vi "Get Target Branch Names.vi"(8 "error in":errorcluster, 11 "Peer Review in":refnum<class "Peer Review.lvclass">) -> (0 "error out":errorcluster, 3 "Peer Review out":refnum<class "Peer Review.lvclass">)   [LabVIEW 2020, in "Peer Review.lvclass"]
uses:
  Peer Review.lvclass
  Peer Review.lvclass/Peer Review.ctl
  <vilib>/Utility/error.llb/Trim Whitespace One-Sided.vi
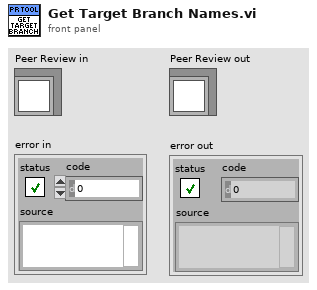
[diagram p1: front panel]
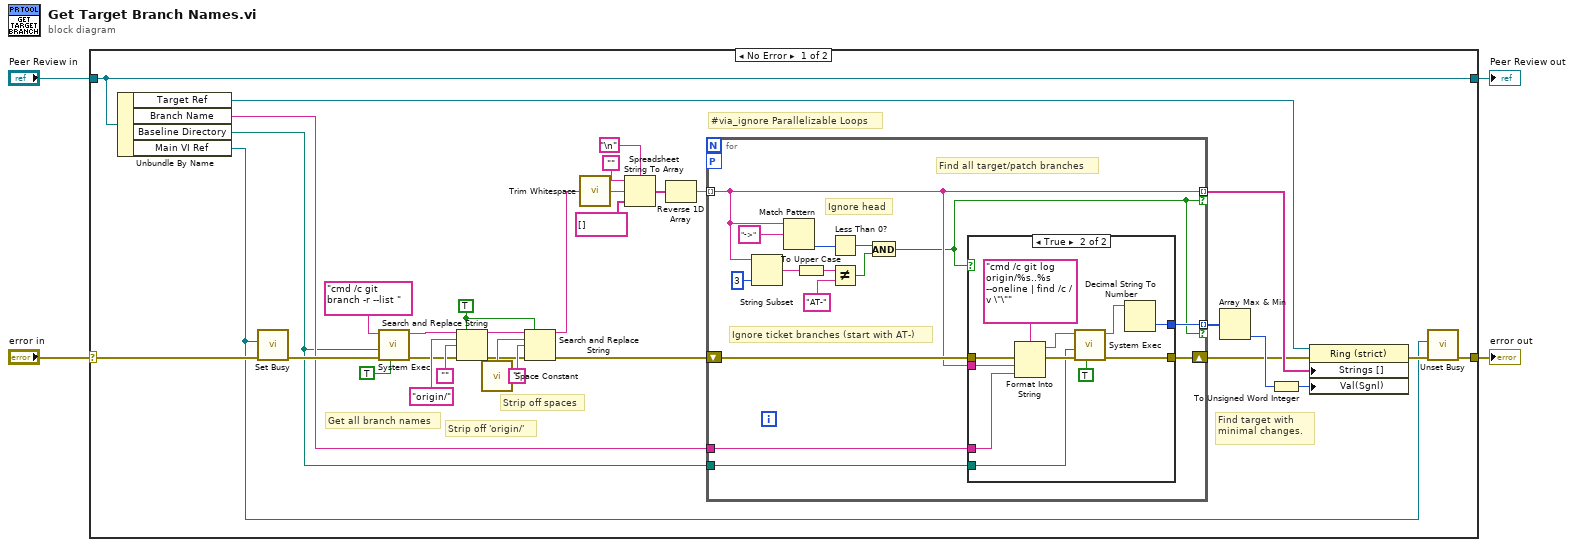
[diagram p0: block diagram]
diagram:
  n1 = case shown="No Error" "error in" {
    selector: "error in" -> [w33 w65]
    tunnel: [w31 w65] -> w3
    tunnel: [w37 w66] -> w4
    tunnel: "Peer Review in" -> [w37 w66]
    frame No Error {
      w11 = TRUE ("replace all? (F)")
      # "#via_ignore Parallelizable Loops"
      # "Find target with minimal changes."
      # "Strip off spaces"
      # "Strip off 'origin/'"
      # "Get all branch names"
      n2 = Unbundle By Name(w37) -> ("Target Ref"=w36:refnum<vi>, "Branch Name"=w8:string, "Baseline Directory"=w7:path, "Main VI Ref"=w10:refnum<vi>)
      n3 = call <vilib>:"Set Busy.vi"("error in (no error)"=w33, "VI reference (current VI)"=w10) -> ("error out"=w13:errorcluster)  [unwired: 8 in, 1 out]
      n4 = call <vilib>:"System Exec.vi"("run minimized? (F)"=TRUE, "error in (no error)"=w13, "working directory"=w7, "command line"="cmd /c git branch -r --list " ("String 2")) -> ("error out"=w21:errorcluster, "standard output"=w23:string)  [unwired: 4 in, 2 out]
      n5 = Search and Replace String(replace all?=w11, input string=w23, search string="origin/", replace string="" ("Empty String Constant"), error in=w21) -> (result string=w27:string, error out=w24:errorcluster)  [unwired: 3 in, 2 out]
      n6 = call <vilib>:"Space Constant.vi"() -> ("String"=w25:string)
      n7 = Search and Replace String(replace all?=w11, input string=w27, search string=w25, replace string="" ("Empty String Constant"), error in=w24) -> (result string=w16:string, error out=w9:errorcluster)  [unwired: 3 in, 2 out]
      n8 = call <vilib>:"Trim Whitespace.vi"("string"=w16) -> ("trimmed string"=w17:string)  [unwired: 1 in]
      n9 = Spreadsheet String To Array(delimiter (Tab)="\n" ("Line Feed Constant"), format string="", spreadsheet string=w17, array type (2D Dbl)=string[] [] ("Strings []")) -> (array=w15:string[])
      n10 = Reverse 1D Array(array=w15) -> (reversed array=w14:string[])
      n11 = for {
        tunnel: w14 -> [w40] mode=indexing
        tunnel: [w40] -> w12 mode=indexing if=w38
        workers-P: _ -> [_]
        tunnel: w8 -> [w50]
        tunnel: [w49] -> w6 mode=indexing if=w38
        tunnel: w7 -> [w48]
        shift-right: [w51] -> w5
        shift-left: w9 -> [w52]
        # "Ignore ticket branches (start with AT-)"
        # "Ignore head"
        # "Find all target/patch branches"
        n12 = String Subset(string=w40, length (rest)=3 ("length (rest)")) -> (substring=w44:string)  [unwired: 1 in]
        n13 = Match Pattern(string=w40, regular expression="->") -> (offset past match=w46:i32)  [unwired: 1 in, 3 out]
        n14 = To Upper Case(1:w44) -> (0:w43:string)
        n15 = Less Than 0?(x=w46) -> (x < 0?=w39:bool)
        n16 = Not Equal?(x=w43, y="AT-") -> (x != y?=w42:bool)
        n17 = And(x=w39, y=w42) -> (x .and. y?=w38:bool)
        n18 = case shown="True" w38 {
          tunnel: w52 -> [w53 w60]
          tunnel: [w53 w59] -> w51
          tunnel: w40 -> [_ w58]
          tunnel: w50 -> [_ w57]
          tunnel: [_ w54] -> w49
          tunnel: w48 -> [_ w55]
          frame False {
          }
          frame True {
            n19 = Format Into String(format string="cmd /c git log origin/%s..%s --oneline | find /c /v \"\"" ("String 2"), error in=w60, w58, w57) -> (resulting string=w63:string, error out=w61:errorcluster)  [unwired: 1 in]
            n20 = call <vilib>:"System Exec.vi"("run minimized? (F)"=TRUE, "error in (no error)"=w61, "working directory"=w55, "command line"=w63) -> ("error out"=w59:errorcluster, "standard output"=w56:string)  [unwired: 4 in, 2 out]
            n21 = Decimal String To Number(string=w56) -> (number=w54:i32)  [unwired: 2 in, 1 out]
          }
        }
      }
      n22 = Array Max & Min(array=w6) -> (min index (indices)=w35:i32)  [unwired: 3 out]
      n23 = To Unsigned Word Integer(number=w35) -> (unsigned 16bit integer=w34:u16)
      n24 = property on="Property Node" class="Ring (strict)"(reference=w36, error in=w5, "Strings []"=w12, "Val(Sgnl)"=w34) -> (error out=w32:errorcluster)  [unwired: 1 out]
      n25 = call <vilib>:"Unset Busy.vi"("error in (no error)"=w32, "VI reference (current VI)"=w10) -> ("error out"=w31:errorcluster)  [unwired: 9 in]
    }
    frame Error {
    }
  }
  "error out" <- w3
  "Peer Review out" <- w4
